vi "Reposition Wheels on Steering Frame.vi"   [LabVIEW 2017, in "NI_Robotics_Steering Frame.lvclass"]
doc: "Changes the location of the wheel or wheels to the position and angle you specify. You must manually select the polymorphic instance to use."
uses:
  <vilib>/robotics/Steering/Steering Frame/NI_Robotics_Steering Frame.lvclass
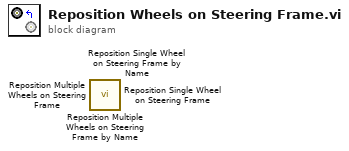
[diagram p0: block diagram]
diagram:
  n1 = call <vilib>:"Reposition Multiple Wheels on Steering Frame by Name.vi"() -> ()  [unwired: 9 in, 3 out]
  n2 = call <vilib>:"Reposition Single Wheel on Steering Frame by Name.vi"() -> ()  [unwired: 9 in, 3 out]
  n3 = call <vilib>:"Reposition Multiple Wheels on Steering Frame.vi"() -> ()  [unwired: 9 in, 3 out]
  n4 = call <vilib>:"Reposition Single Wheel on Steering Frame.vi"() -> ()  [unwired: 9 in, 3 out]
